vi "Modbus Convert to Blower Pressure.vi"(11 "Blower Voltage Output (mV)":i16) -> (3 "Blower Pressure (in. W.C)":dbl)   [LabVIEW 2023, in "Modbus.lvlib"]
uses:
  Modbus.lvlib
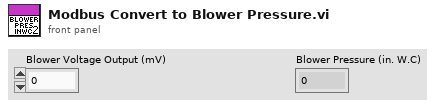
[diagram p1: front panel]
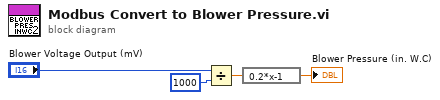
[diagram p0: block diagram]
diagram:
  n1 = Divide(x="Blower Voltage Output (mV)", y=i16 1000) -> (x/y=w2:dbl)
  n2 = expression code="0.2*x-1"(w2) -> (→"Blower Pressure (in. W.C)":dbl)
